vi "Test_LogValueEvent_LogStr_MatchFormattoString.vi"(8 "error in (no error)":errorcluster, 11 "TestCase in":refnum<class "TestLogValue.lvclass">) -> (0 "error out":errorcluster, 3 "TestCase out":refnum<class "TestLogValue.lvclass">)   [LabVIEW 2019, in "TestLogValue.lvclass"]
uses:
  TestLogValue.lvclass
  Source/Composed Log/Types/Log Level.ctl
  Source/Composed Log/LoggerReference/LoggerReference.lvclass/LoggerReference.ctl
  Source/LVQueue Sink/LVQueue Sink.lvclass/LVQueue Sink.ctl
  272d61b2-f49c-486c-9daf-337ffb054b40.vi
  154dbc8a-62f5-4aa1-ad82-2a3c469f95b7.vi
  Source/Composed Log/LoggerReference/Return Aggregate Queues.vi
  Source/Composed Log/LoggerReference/Add Aggregate Log.vi
  272d61b2-f49c-486c-9daf-337ffb054b40.vi/bce8171a-b0d5-45d7-8f54-bef9982cf948.vi
  154dbc8a-62f5-4aa1-ad82-2a3c469f95b7.vi/7940ba36-9a42-4057-8e93-c09e8a570659.vi
  Source/Composed Log/LoggerReference/Get Valid Event Time.vi
  Source/Composed Log/LoggerReference/Log Event.vi
  Source/Composed Log/LoggerReference/Send Add Sink.vi
  Source/Composed Log/LoggerReference/Log.vi
  Source/Composed Log/LoggerReference/Remove Stale Logs.vi
  Source/LVQueue Sink/LVQueue Sink.lvclass
  C:/CS/Log/Source/Composed Log/Log Sink/Log Sink.lvclass
  Source/Composed Log/Application Logger/Launch Worker Loop.vi
  Source/Composed Log/LoggerReference/Initialize Logger Instance.vi
  Source/Composed Log/LoggerReference/LoggerReference.lvclass
  Source/Composed Log/IErrorFormat/IErrorFormat.lvclass
  Source/Composed Log/Log Sink/Log Sink.lvclass
  <vilib>/addons/_JKI Toolkits/VI Tester/TestCase.llb/TestCase.lvclass
  Source/Composed Log/Composed Log.lvlib
  C:/Program Files (x86)/National Instruments/LabVIEW 2019/vi.lib/addons/_JKI Toolkits/VI Tester/TestCase.llb/TestCase.lvclass
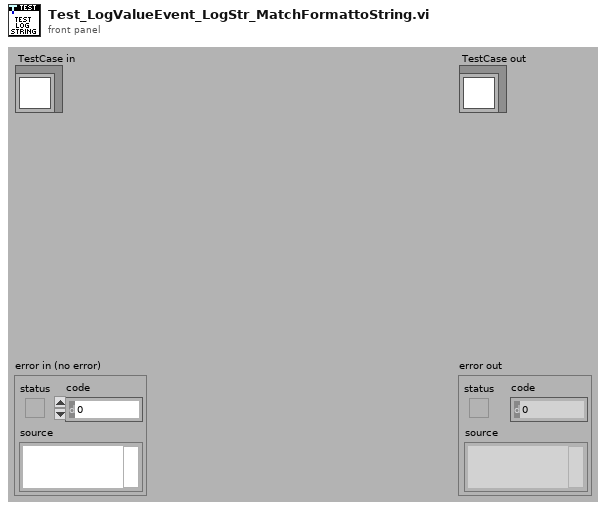
[diagram p1: front panel]
types:
  T1 = typedef "Composed Log.lvlib/Log Level.ctl" = enum16{"Debug", "Info", "Warning", "Error", "Critical"}
  T2 = typedef "Composed Log.lvlib/Log Packet.ctl" = cluster{"Data To Log":string, "Source":string, "Event Level":T1, "Event Time":timestamp}
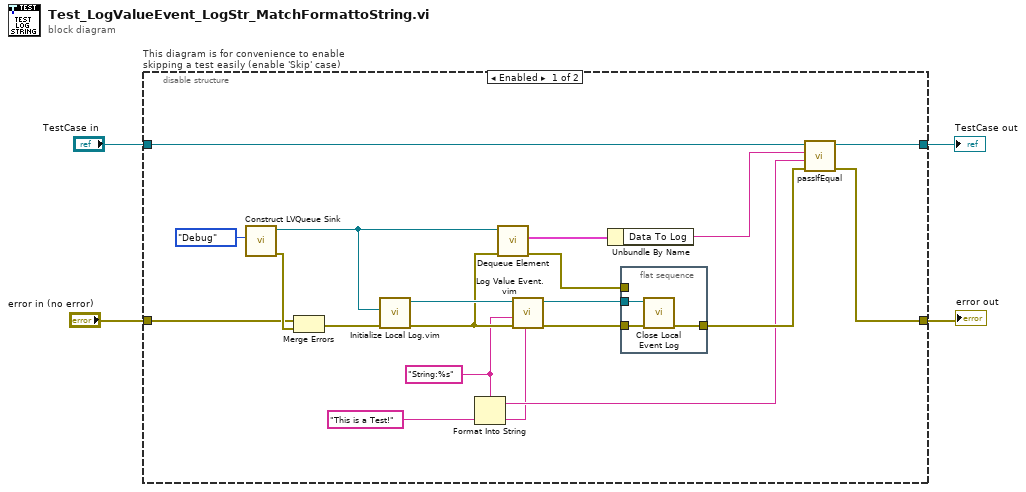
[diagram p0: block diagram]
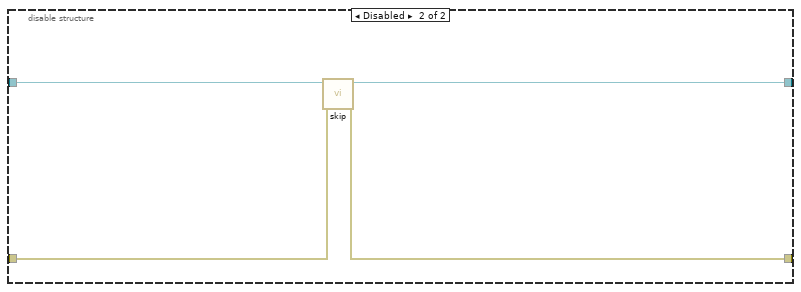
[diagram p2: hidden frame]
diagram:
  n1 = disable-structure "This diagram is for convenience to enable skipping a test easily (enable 'Skip' case)" shown="Enabled" {
    disable-tunnel: "TestCase in" -> [w17 w30]
    disable-tunnel: [w16 w28] -> w1
    disable-tunnel: [w14 w29] -> w3
    disable-tunnel: "error in (no error)" -> [w15 w27]
    frame Enabled {
      w5 = "This is a Test!"
      w9 = "String:%s" ("Data To Log")
      n2 = call "Construct LVQueue Sink.vi"("LogLevel"=Log_Level."Debug") -> ("error out"=w20:errorcluster, "LVQueue Sink out"=w18:refnum<class "LVQueue Sink.lvclass">)  [unwired: 9 in]
      n3 = Merge Errors(w15, w20) -> (w19:errorcluster)
      n4 = call "Initialize Local Log.vim"("error in (no error)"=w19, "Startup Sink(s)"=w18) -> ("error out"=w12:errorcluster, "Log Instance Reference"=w13:refnum<class "LoggerReference.lvclass">)  [unwired: 7 in, 1 out]
      n5 = Format Into String(format string=w9, w5) -> (resulting string=w7:string)  [unwired: 2 in, 1 out]
      n6 = call "Dequeue Element.vi"("error in (no error)"=w12, "LVQueue Sink in"=w18) -> ("error out"=w23:errorcluster, "Log Packet"=w21:T2)  [unwired: 6 in, 2 out]
      n7 = call "Log Value Event.vim"("Value(s)"=w5, "error in (no error)"=w12, "Log Message Format String"=w9, "LoggerReference in"=w13) -> ("error out"=w11:errorcluster, "LoggerReference out"=w10:refnum<class "LoggerReference.lvclass">)  [unwired: 6 in]
      n8 = Unbundle By Name(w21) -> ("Data To Log"=w8:string)
      n9 = flat-sequence {
        tunnel: [w25] -> w22
        tunnel: w11 -> [w26]
        tunnel: w23 -> [_]
        tunnel: w10 -> [w24]
        frame #0 {
          n10 = call "Close Local Event Log.vi"("error in (no error)"=w26, "Log Instance"=w24) -> ("error out"=w25:errorcluster)  [unwired: 9 in]
        }
      }
      n11 = call-dynamic "passIfEqual.vi"("error in (no error)"=w22, "y"=w7, "x"=w8, "TestCase in"=w17) -> ("error out"=w14:errorcluster, "TestCase out"=w16:refnum<class "TestLogValue.lvclass">)  [unwired: 6 in]
    }
    frame Disabled {
      # "skip test result while test is under development"
      n12 = call <vilib>:"skip.vi"("error in (no error)"=w27, "TestCase in"=w30) -> ("error out"=w29:errorcluster, "TestCase out"=w28:refnum<class "TestLogValue.lvclass">)  [unwired: 8 in]
    }
  }
  "error out" <- w3
  "TestCase out" <- w1
